vi "Error_SubVi.vi"(11 "string":string="FPSP0RP0FS0TL0PP50%TD1000 KmFEBL1CL0RL1FL0AL1HL1G3") -> (3 "error":bool)   [LabVIEW 2014]
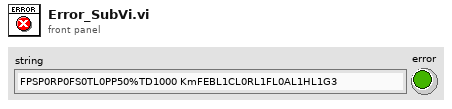
[diagram p1: front panel]
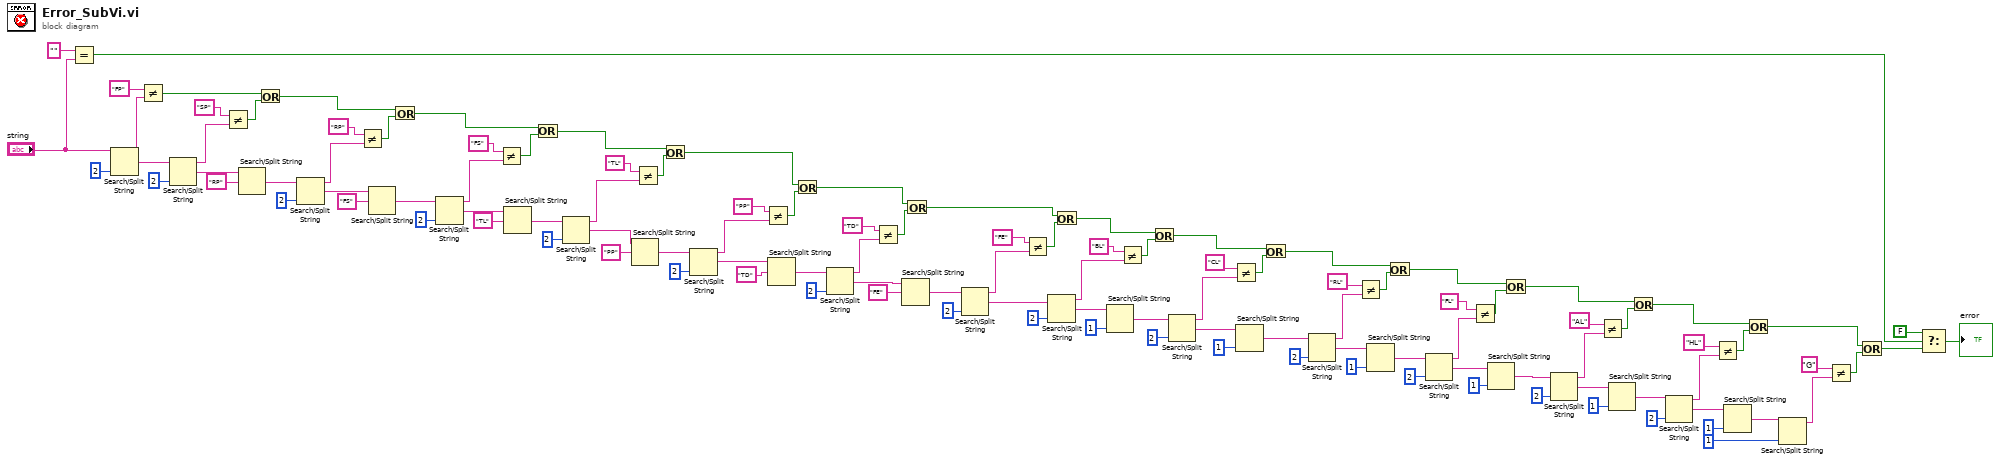
[diagram p0: block diagram]
diagram:
  n1 = Equal?(x="", y="string") -> (x = y?=w39:bool)
  n2 = Search/Split String(string="string", offset (0)=2) -> (substring before match=w98:string, match + rest of string=w71:string)  [unwired: 1 in, 1 out]
  n3 = Not Equal?(x="FP", y=w98) -> (x != y?=w42:bool)
  n4 = Search/Split String(string=w71, offset (0)=2) -> (substring before match=w73:string, match + rest of string=w60:string)  [unwired: 1 in, 1 out]
  n5 = Not Equal?(x="SP", y=w73) -> (x != y?=w100:bool)
  n6 = Search/Split String(string=w60, search string/char (-)="RP") -> (match + rest of string=w62:string)  [unwired: 1 in, 2 out]
  n7 = Or(x=w42, y=w100) -> (x .or. y?=w102:bool)
  n8 = Search/Split String(string=w62, offset (0)=2) -> (substring before match=w75:string, match + rest of string=w64:string)  [unwired: 1 in, 1 out]
  n9 = Not Equal?(x="RP", y=w75) -> (x != y?=w101:bool)
  n10 = Search/Split String(string=w64, search string/char (-)="FS") -> (match + rest of string=w65:string)  [unwired: 1 in, 2 out]
  n11 = Or(x=w102, y=w101) -> (x .or. y?=w104:bool)
  n12 = Search/Split String(string=w65, offset (0)=2) -> (substring before match=w77:string, match + rest of string=w67:string)  [unwired: 1 in, 1 out]
  n13 = Not Equal?(x="FS", y=w77) -> (x != y?=w103:bool)
  n14 = Search/Split String(string=w67, search string/char (-)="TL") -> (match + rest of string=w69:string)  [unwired: 1 in, 2 out]
  n15 = Or(x=w104, y=w103) -> (x .or. y?=w106:bool)
  n16 = Search/Split String(string=w69, offset (0)=2) -> (substring before match=w79:string, match + rest of string=w28:string)  [unwired: 1 in, 1 out]
  n17 = Search/Split String(string=w28, search string/char (-)="PP") -> (match + rest of string=w31:string)  [unwired: 1 in, 2 out]
  n18 = Not Equal?(x="TL", y=w79) -> (x != y?=w105:bool)
  n19 = Or(x=w106, y=w105) -> (x .or. y?=w26:bool)
  n20 = Search/Split String(string=w31, offset (0)=2) -> (substring before match=w27:string, match + rest of string=w24:string)  [unwired: 1 in, 1 out]
  n21 = Not Equal?(x="PP", y=w27) -> (x != y?=w30:bool)
  n22 = Search/Split String(string=w24, search string/char (-)="TD") -> (match + rest of string=w36:string)  [unwired: 1 in, 2 out]
  n23 = Or(x=w26, y=w30) -> (x .or. y?=w22:bool)
  n24 = Search/Split String(string=w36, offset (0)=2) -> (substring before match=w25:string, match + rest of string=w20:string)  [unwired: 1 in, 1 out]
  n25 = Not Equal?(x="TD", y=w25) -> (x != y?=w37:bool)
  n26 = Search/Split String(string=w20, search string/char (-)="FE") -> (match + rest of string=w4:string)  [unwired: 1 in, 2 out]
  n27 = Or(x=w22, y=w37) -> (x .or. y?=w23:bool)
  n28 = Search/Split String(string=w4, offset (0)=2) -> (substring before match=w2:string, match + rest of string=w1:string)  [unwired: 1 in, 1 out]
  n29 = Not Equal?(x="FE", y=w2) -> (x != y?=w107:bool)
  n30 = Search/Split String(string=w1, offset (0)=2) -> (substring before match=w82:string, match + rest of string=w56:string)  [unwired: 1 in, 1 out]
  n31 = Or(x=w23, y=w107) -> (x .or. y?=w109:bool)
  n32 = Search/Split String(string=w56, offset (0)=1) -> (match + rest of string=w50:string)  [unwired: 1 in, 2 out]
  n33 = Not Equal?(x="BL", y=w82) -> (x != y?=w108:bool)
  n34 = Or(x=w109, y=w108) -> (x .or. y?=w111:bool)
  n35 = Search/Split String(string=w50, offset (0)=2) -> (substring before match=w84:string, match + rest of string=w53:string)  [unwired: 1 in, 1 out]
  n36 = Not Equal?(x="CL", y=w84) -> (x != y?=w110:bool)
  n37 = Search/Split String(string=w53, offset (0)=1) -> (match + rest of string=w51:string)  [unwired: 1 in, 2 out]
  n38 = Or(x=w111, y=w110) -> (x .or. y?=w113:bool)
  n39 = Search/Split String(string=w51, offset (0)=2) -> (substring before match=w86:string, match + rest of string=w48:string)  [unwired: 1 in, 1 out]
  n40 = Not Equal?(x="RL", y=w86) -> (x != y?=w112:bool)
  n41 = Search/Split String(string=w48, offset (0)=1) -> (match + rest of string=w46:string)  [unwired: 1 in, 2 out]
  n42 = Or(x=w113, y=w112) -> (x .or. y?=w115:bool)
  n43 = Search/Split String(string=w46, offset (0)=2) -> (substring before match=w88:string, match + rest of string=w94:string)  [unwired: 1 in, 1 out]
  n44 = Not Equal?(x="FL", y=w88) -> (x != y?=w114:bool)
  n45 = Search/Split String(string=w94, offset (0)=1) -> (match + rest of string=w96:string)  [unwired: 1 in, 2 out]
  n46 = Or(x=w115, y=w114) -> (x .or. y?=w117:bool)
  n47 = Search/Split String(string=w96, offset (0)=2) -> (substring before match=w90:string, match + rest of string=w92:string)  [unwired: 1 in, 1 out]
  n48 = Not Equal?(x="AL", y=w90) -> (x != y?=w116:bool)
  n49 = Search/Split String(string=w92, offset (0)=1) -> (match + rest of string=w13:string)  [unwired: 1 in, 2 out]
  n50 = Or(x=w117, y=w116) -> (x .or. y?=w12:bool)
  n51 = Search/Split String(string=w13, offset (0)=2) -> (substring before match=w19:string, match + rest of string=w17:string)  [unwired: 1 in, 1 out]
  n52 = Not Equal?(x="HL", y=w19) -> (x != y?=w14:bool)
  n53 = Search/Split String(string=w17, offset (0)=1) -> (match + rest of string=w5:string)  [unwired: 1 in, 2 out]
  n54 = Or(x=w12, y=w14) -> (x .or. y?=w7:bool)
  n55 = Search/Split String(string=w5, offset (0)=1) -> (substring before match=w8:string)  [unwired: 1 in, 2 out]
  n56 = Not Equal?(x="G", y=w8) -> (x != y?=w11:bool)
  n57 = Or(x=w7, y=w11) -> (x .or. y?=w6:bool)
  n58 = Select(t=FALSE, s=w39, f=w6) -> (s? t:f=→"error":bool)
